vi "Close semaphore.vi"(8 "error in (no error)":errorcluster, 11 "semaphore":T1) -> (0 "error out":errorcluster, 3 "semaphore name":string)   [LabVIEW 2014, in "Simatic S7.lvlib"]
uses:
  Simatic S7.lvlib
panel:
  # "Release Semaphore Reference.vi<APPEND>\n\n<b>Complete call chain:</b>\n     Release Semaphore Reference.vi\n     Simatic S7.lvlib:Close semaphore.vi\n     Simatic S7.lvlib:Global PLC Ref.vi"
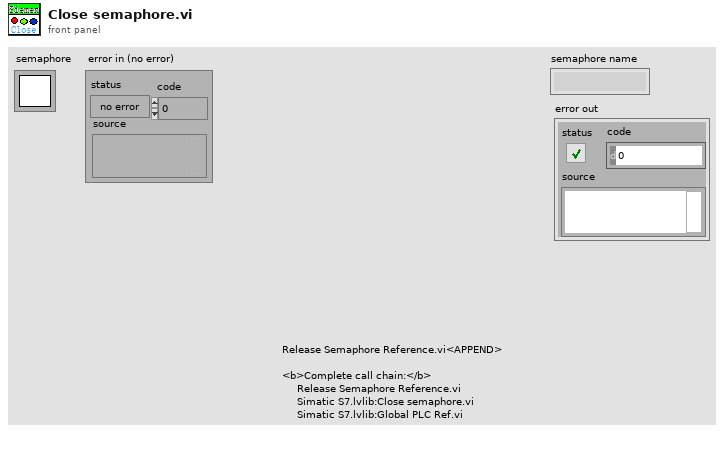
[diagram p1: front panel]
types:
  T1 = typedef "Semaphore RefNum" = refnum<k1>
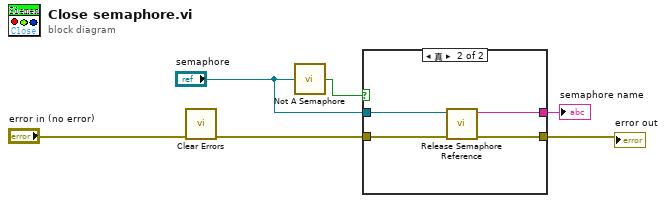
[diagram p0: block diagram]
diagram:
  n1 = call <vilib>:"Clear Errors.vi"("error in (no error)"="error in (no error)") -> ("error out"=w5:errorcluster)  [unwired: 5 in, 1 out]
  n2 = call <vilib>:"Not A Semaphore.vi"("semaphore"="semaphore") -> ("not a semaphore"=w4:bool)
  n3 = case shown="真" w4 {
    tunnel: w5 -> [w7 w9]
    tunnel: [w7 w11] -> w2
    tunnel: [_ w10] -> w3
    tunnel: "semaphore" -> [_ w8]
    frame False {
    }
    frame True {
      n4 = call <vilib>:"Release Semaphore Reference.vi"("error in (no error)"=w9, "semaphore"=w8) -> ("error out"=w11:errorcluster, "semaphore name"=w10:string)  [unwired: 8 in]
    }
  }
  "semaphore name" <- w3
  "error out" <- w2
